vi "VINameToControls.vi"(7 "application reference (local)":refnum<vi>, 8 "error in (no error)":errorcluster, 10 "vi ref":refnum<vi>, 11 "vi":string) -> (0 "error out":errorcluster, 3 "FlattenControls[]":refnum<vi>[](array[refnum]), 5 "VI out":refnum<vi>)   [LabVIEW 2019]
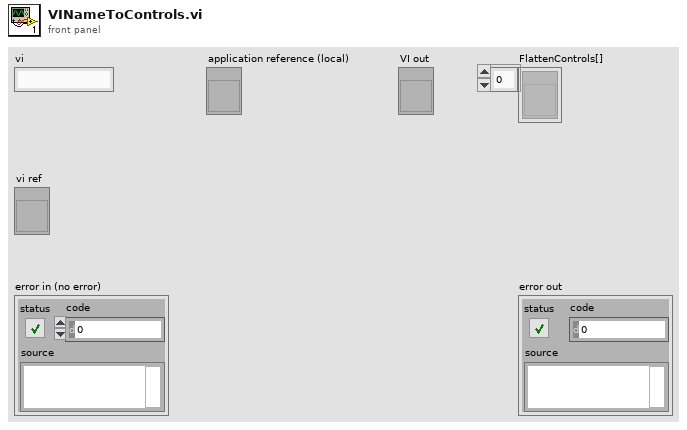
[diagram p1: front panel]
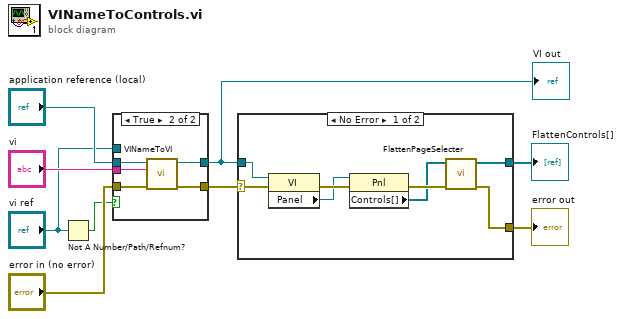
[diagram p0: block diagram]
diagram:
  n1 = Not A Number/Path/Refnum?(number/path/refnum="vi ref") -> (NaN/Path/Refnum?=w2:bool)
  n2 = case shown="True" w2 {
    tunnel: [w10 w16] -> w9
    tunnel: "vi" -> [_ w15]
    tunnel: "error in (no error)" -> [w11 w14]
    tunnel: "application reference (local)" -> [_ w13]
    tunnel: [w11 w12] -> w3
    tunnel: "vi ref" -> [w10 _]
    frame False {
    }
    frame True {
      n3 = call "VINameToVI.vi"("error in (no error)"=w14, "vi"=w15, "Application in"=w13) -> ("error out"=w12:errorcluster, "VI out"=w16:refnum<vi>)  [unwired: 7 in]
    }
  }
  "VI out" <- w9
  n4 = case shown="No Error" w3 {
    selector: w3 -> [w17 w25]
    tunnel: w9 -> [w24 _]
    tunnel: [w23 w25] -> w6
    tunnel: [w21 _] -> w5
    frame No Error {
      n5 = property class="VI"(reference=w24, error in=w17) -> (error out=w19:errorcluster, "Panel"=w18:refnum<vi>)  [unwired: 1 out]
      n6 = property class="Pnl"(reference=w18, error in=w19) -> (error out=w22:errorcluster, "Controls[]"=w20:refnum<vi>[])  [unwired: 1 out]
      n7 = call "FlattenPageSelecter.vi"("error in (no error)"=w22, "Controls[]"=w20) -> ("error out"=w23:errorcluster, "Flatten[]"=w21:refnum<vi>[])  [unwired: 8 in]
    }
    frame Error {
    }
  }
  "error out" <- w6
  "FlattenControls[]" <- w5
